vi "NearFieldCamera_param.vi"() -> ()   [LabVIEW 2018]
panel:
  in  "曝光时间/us":dbl=100.0 min=100.0
  in  "模拟增益/dB":u64=8 min=8
  in  "相机IP":string="192.168.129.10"
  # "近场相机\n参数"
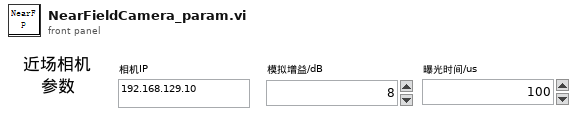
[diagram p1: front panel]
types:
  T1 = typedef "Image Type" = u32
  T2 = typedef "IMAQ Image.ctl" = refnum<image>
  T3 = cluster{"示波器":cluster{"Channel (0:Channel 1)":enum16{"Channel 1", "Channel 2", "Channel 3", "Channel 4"}, "电压范围":dbl, "触发电压":dbl, "时间范围":dbl, " 示波器VISA":refnum<visa-resource-name>, "时间范围 标签":u64, "电压范围 标签":u64, "触发电压 标签":u64, "输入阻抗/Ω":u64}, "光谱仪":cluster{"SpecDataReference":refnum<queue>, "grating center":dbl, "Exposure Time (s)":dbl, "是否进行详细设置":bool, " 开始通信检查":bool, "通信成功？":bool, "波长":dbl}, " 近场相机":cluster{"曝光时间/100us":dbl, "模拟增益":i32, "控制套接字":i32, "IP 地址":string, " 采集套接字":i32, "  版本号":i32, "ImageData":T2, "  增益最大":i32, "  增益最小":i32, " 曝光最大":i32, " 曝光最小":i32, " 帧速":i32, " 同步切换":i32, "  曝光缩放":i32}, " 偏振仪":cluster{"电压范围":u64, "触发电压":u64, "时间范围":u64, "波长范围":enum16{"可见光 400-700nm", "近红外 700-1100nm"}, "可见光偏振测量仪VISA":refnum<visa-resource-name>, "近红外偏振测量仪VISA":refnum<visa-resource-name>}, " 功率计":cluster{"通道":enum16{"Channel 1", "Channel 2"}, "工作波长":u32, "单位":u64, "时间范围":u64, "IP地址":string, "端口":u32}, "能量计":cluster{"通道":enum16{"Channel 1", "Channel 2"}, "工作波长":u32, "单位":u64, "时间范围":u64, "IP地址":string, "端口":u32, "能量计量程":enum16{"200uJ", "20uJ", "2uJ", "200nJ"}}, "电机":cluster{"Channel (0:Channel 1)":enum16{"Channel 1", "Channel 2", "Channel 3", "Channel 4"}, "电压范围":u64, "触发电压":u64, "时间范围":u64}, " 远场相机":cluster{"曝光时间":i32, "模拟增益":i32, "控制套接字":i32, "IP 地址":string, " 采集套接字":i32, "  版本号":i32, "ImageData":T2, "  增益最大":i32, "  增益最小":i32, " 曝光最大":i32, " 曝光最小":i32, " 帧速":i32, " 同步切换":i32, "  曝光缩放":i32, "ImageData B":T2}}
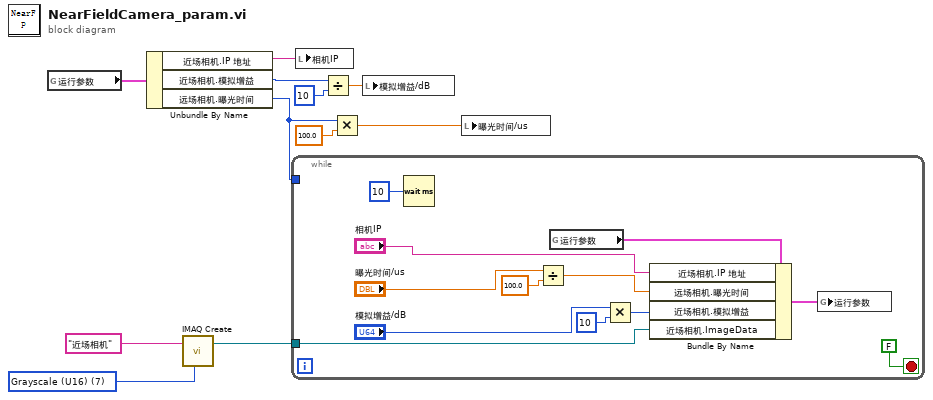
[diagram p0: block diagram]
diagram:
  w10 = T1 7 items=["Grayscale (U8)", "Grayscale (I16)", "Grayscale (SGL)", "Complex (CSG)", "RGB (U32)", "HSL (U32)", "RGB (U64)", "Grayscale (U16)"] ("Image Type")
  n1 = global read "参数.vi" "运行参数"() -> (w8:T3)
  n2 = Unbundle By Name(w8) -> ("近场相机.IP 地址"=w7:string, "近场相机.模拟增益"=w3:i32, "远场相机.曝光时间"=w6:i32)
  n3 = call "IMAQ Create"("Image Name"="近场相机", "Image Type"=w10) -> ("New Image"=w9:T2)  [unwired: 3 in, 1 out]
  n4 = while {
    tunnel: w9 -> [w18]
    tunnel: w6 -> [_]
    stop <- FALSE stop-if-true
    n5 = Wait (ms)(milliseconds to wait=u32 10 ("等待时间（毫秒）")) -> ()  [unwired: 1 out]
    n6 = Divide(x="曝光时间/us", y=100.0) -> (x/y=w15:dbl)
    n7 = global read "参数.vi" "运行参数"() -> (w21:T3)
    n8 = Multiply(x="模拟增益/dB", y=u64 10) -> (x*y=w12:u64)
    n9 = Bundle By Name(cluster=w21, "近场相机.IP 地址"="相机IP", "远场相机.曝光时间"=w15, "近场相机.模拟增益"=w12, "近场相机.ImageData"=w18) -> (w19:T3)
    n10 = global write "参数.vi" "运行参数"(w19) -> ()
  }
  n11 = local write "相机IP"(w7) -> ()
  n12 = Divide(x=w3, y=10) -> (x/y=w1:dbl)
  n13 = Multiply(x=w6, y=100.0) -> (x*y=w4:dbl)
  n14 = local write "模拟增益/dB"(w1) -> ()
  n15 = local write "曝光时间/us"(w4) -> ()
